vi "GetPhaseBandWaveform.vi"(4 "source channel wfm":waveform(sgl), 6 "source channel wfm found":bool, 8 "error in (no error)":errorcluster, 9 "waveform":waveform(sgl), 10 "channel":T1, 11 "all waveforms":waveform(sgl)[](array[waveform])) -> (0 "error out":errorcluster, 1 "channel name of waveform to use in phase band calculation":string, 2 "conversion op":T5, 3 "waveform to use in phase band calculation":waveform(sgl))   [LabVIEW 2017, in "AnalysisHelper.lvlib"]
uses:
  <vilib>/addons/InsightCM/Utilities/Analysis/Shared/AnalysisHelper.lvlib
  <vilib>/addons/InsightCM/Utilities/Analysis/Shared/controls/ConversionOp.ctl
  <vilib>/addons/InsightCM/Utilities/Analysis/Shared/controls/Channel.ctl
  <vilib>/addons/InsightCM/Utilities/Analysis/Shared/controls/SpeedType.ctl
  <vilib>/addons/InsightCM/Utilities/Analysis/Shared/controls/Feature.ctl
  <vilib>/addons/InsightCM/Utilities/Analysis/Shared/controls/AmplitudeScale.ctl
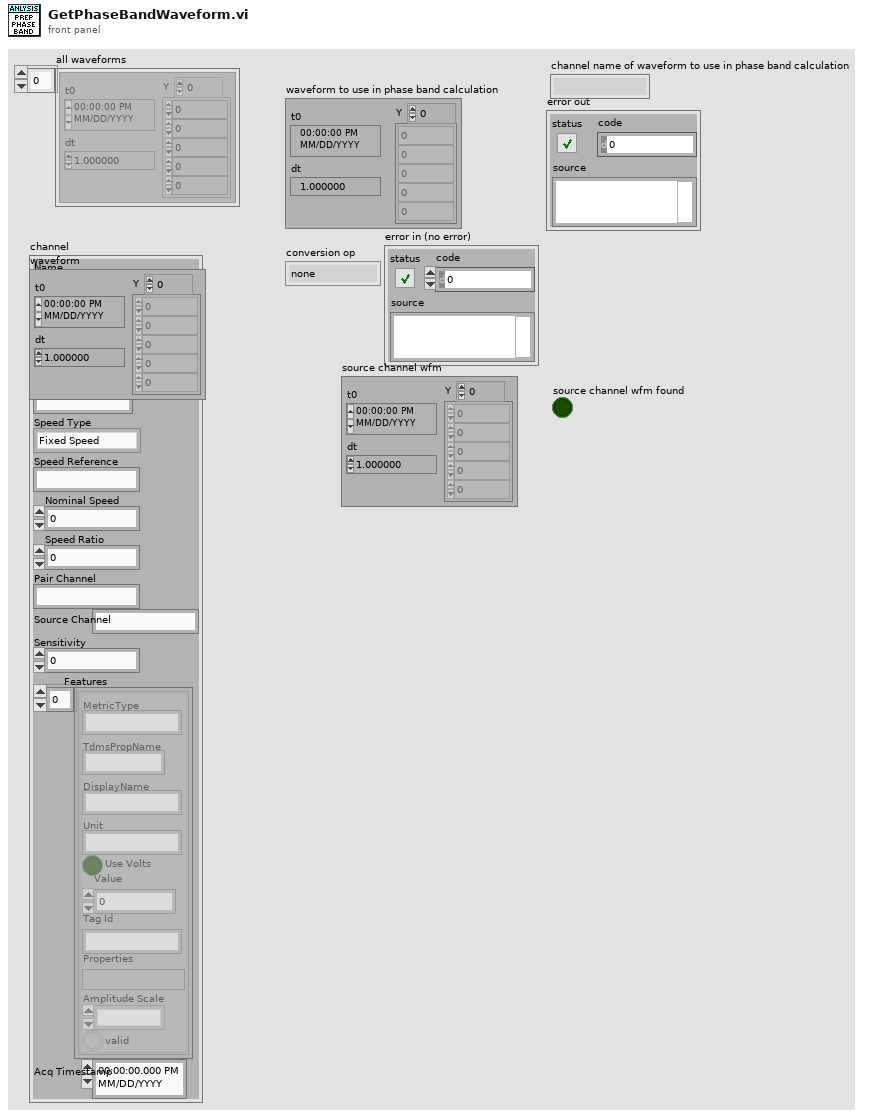
[diagram p1: front panel]
types:
  T1 = typedef "AnalysisHelper.lvlib/Channel.ctl" = cluster{"Name":string, "Id":string, "Type":string, "Status Tag":string, "Speed Type":T2, "Speed Reference":string, "Nominal Speed":dbl, "Speed Ratio":dbl, "Pair Channel":string, "Source Channel":string, "Sensitivity":dbl, "Features":T3[], "Acq Timestamp":timestamp}
  T2 = typedef "AnalysisHelper.lvlib/SpeedType.ctl" = enum16{"Fixed Speed", "Tachometer"}
  T3 = typedef "AnalysisHelper.lvlib/Feature.ctl" = cluster{"MetricType":string, "TdmsPropName":string, "DisplayName":string, "Unit":string, "Use Volts":bool, "Value":dbl, "Tag Id":string, "Properties":variant, "Amplitude Scale":T4, "valid":bool}
  T4 = typedef "AnalysisHelper.lvlib/AmplitudeScale.ctl" = enum16{"rms", "peak", "pk-pk"}
  T5 = typedef "AnalysisHelper.lvlib/ConversionOp.ctl" = enum16{"none", "singleInt", "doubleInt", "singleDiff", "doubleDiff"}
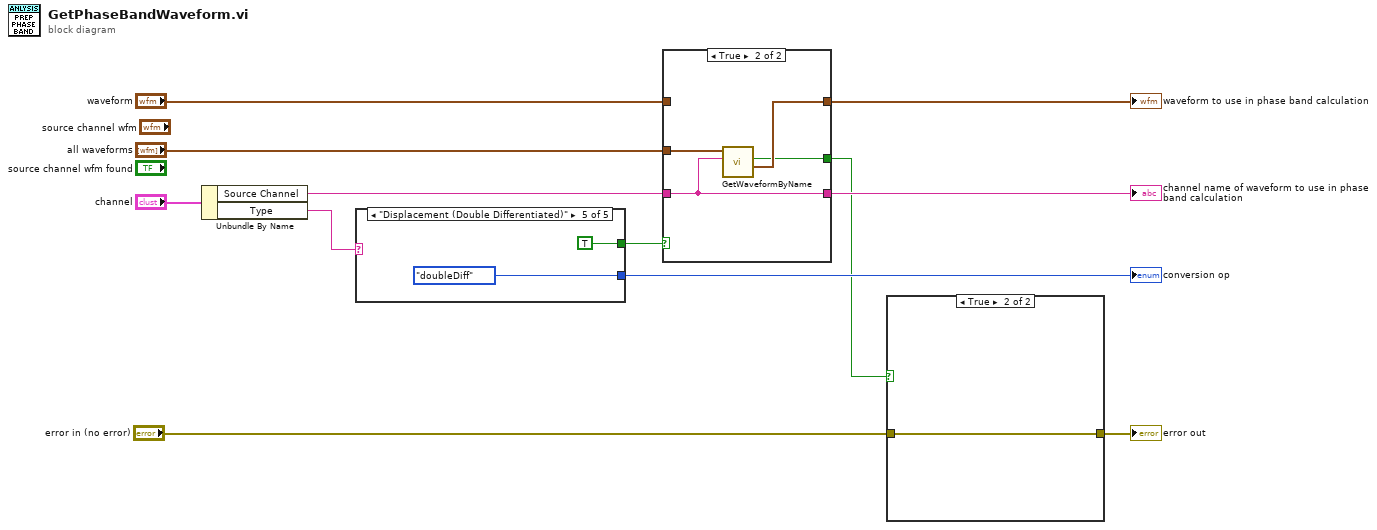
[diagram p0: block diagram]
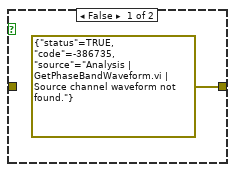
[diagram p2: hidden frame]
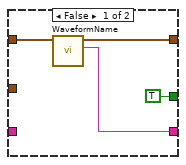
[diagram p3: hidden frame]
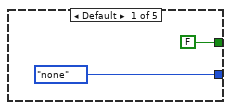
[diagram p4: hidden frame]
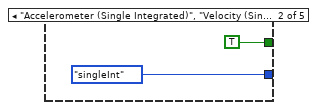
[diagram p5: hidden frame]
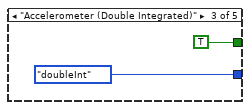
[diagram p6: hidden frame]
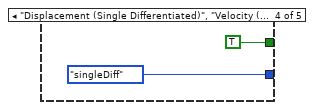
[diagram p7: hidden frame]
diagram:
  n1 = Unbundle By Name("channel") -> ("Source Channel"=w6:string, "Type"=w12:string)
  n2 = case shown="\"Displacement (Double Differentiated)\"" w12 {
    tunnel: [ConversionOp."none" ("Conversion Op (phase sb only)") ConversionOp."singleInt" ("Conversion Op (phase sb only)") ConversionOp."doubleInt" ("Conversion Op (phase sb only)") ConversionOp."singleDiff" ("Conversion Op (phase sb only)") ConversionOp."doubleDiff" ("Conversion Op (phase sb only)")] -> w10
    tunnel: [FALSE TRUE TRUE TRUE TRUE] -> w9
    frame Default {
    }
    frame "Accelerometer (Single Integrated)", "Velocity (Single Integrated)" {
    }
    frame "Accelerometer (Double Integrated)" {
    }
    frame "Displacement (Single Differentiated)", "Velocity (Single Differentiated)" {
    }
    frame "Displacement (Double Differentiated)" {
    }
  }
  "conversion op" <- w10
  n3 = case shown="True" w9 {
    tunnel: [w24 w28] -> w8
    tunnel: "waveform" -> [w25 _]
    tunnel: w6 -> [_ w29]
    tunnel: [w26 w29] -> w5
    tunnel: "all waveforms" -> [_ w30]
    tunnel: [TRUE ("Found?") w27] -> w3
    frame False {
      n4 = call <vilib>:"WaveformName.vi"("signal in"=w25) -> ("name"=w26:string, "signal out"=w24:waveform(sgl))  [unwired: 9 in]
    }
    frame True {
      n5 = call <vilib>:"GetWaveformByName.vi"("Channel Name"=w29, "Acq Waveforms"=w30) -> ("Waveform"=w28:waveform(sgl), "Found?"=w27:bool)  [unwired: 6 in, 2 out]
    }
  }
  "waveform to use in phase band calculation" <- w8
  "channel name of waveform to use in phase band calculation" <- w5
  n6 = case shown="True" w3 {
    tunnel: "error in (no error)" -> [_ w32]
    tunnel: [errorcluster {"status"=TRUE, "code"=-386735, "source"="Analysis | GetPhaseBandWaveform.vi | Source channel waveform not found."} ("error in (no error)") w32] -> w1
    frame False {
    }
    frame True {
    }
  }
  "error out" <- w1
